vi "Labview I2C.vi"() -> ()   [LabVIEW 2011]
uses:
  <vilib>/NXT/Block Support/HWPage.SensorType.ctl
  <vilib>/NXT/Block Support/HWPage.SensorMode.ctl
  <vilib>/NXT/Block Support/NXT_InputPort.ctl
panel:
  out "Success?":bool
  out "Bytes read":u8[](array[numeric])
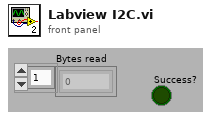
[diagram p1: front panel]
types:
  T1 = typedef "HWPage.SensorType.ctl" = u8
  T2 = typedef "HWPage.SensorMode.ctl" = u8
  T3 = typedef "NXT_InputPort.ctl" = u8
  T4 = typedef "LVHSConnector.ctl" = cluster{"Hardware":string, "Flattened String":string}
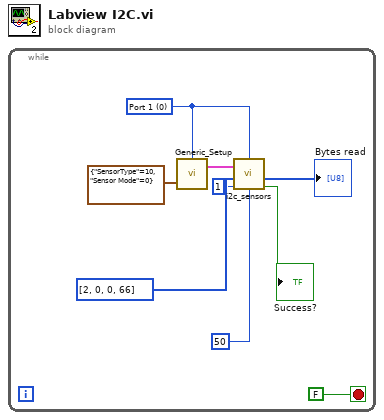
[diagram p0: block diagram]
diagram:
  n1 = while {
    stop <- FALSE stop-if-true
    w5 = T3 0 items=["Port 1", "Port 2", "Port 3", "Port 4"] ("Port")
    n2 = call <vilib>:"Generic_Setup.vi"("Sensor Setup"=cluster{"SensorType":T1, "Sensor Mode":T2} {"SensorType"=10, "Sensor Mode"=0}, "Port"=w5) -> ("NXT"=w9:T4)  [unwired: 1 in, 1 out]
    n3 = call <vilib>:"i2c_sensors.vi"("Return Length"=u8 1, "Bytes to Write"=u8[] [2, 0, 0, 66], "Wait (msec)"=u32 50, "NXT"=w9, "Port"=w5) -> ("Success?"=→"Success?":bool, "Bytes read"=→"Bytes read":u8[])  [unwired: 1 out]
  }
